vi "Read CJC Value.vi"(8 "error in (no error)":errorcluster, 11 "BNT_DMQmx-MCSV-TC in":refnum<class "BNT_DMQmx-MCSV-TC.lvclass">) -> (0 "error out":errorcluster, 2 "CJC Value":dbl=25.0 format="%0.2f", 3 "BNT_DMQmx-MCSV-TC out":refnum<class "BNT_DMQmx-MCSV-TC.lvclass">)   [LabVIEW 2016, in "BNT_DAQmx.lvlib" / "BNT_DMQmx-MCSV-TC.lvclass"]
doc: "Read CJC Value."
uses:
  BNT_DMQmx-MCSV-TC.lvclass
  BNT_DMQmx-MCSV-TC.lvclass/BNT_DMQmx-MCSV-TC.ctl
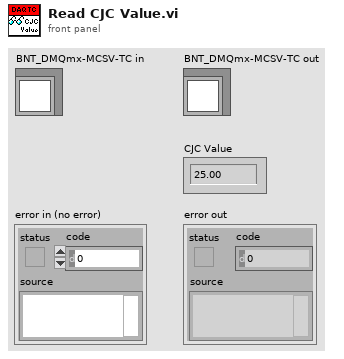
[diagram p1: front panel]
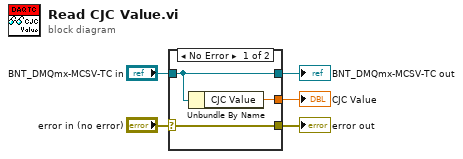
[diagram p0: block diagram]
diagram:
  n1 = case shown="No Error" "error in (no error)" {
    selector: "error in (no error)" -> [w8 w9]
    tunnel: [w8 w9] -> w4
    tunnel: [w7 w10] -> w2
    tunnel: "BNT_DMQmx-MCSV-TC in" -> [w7 w10]
    tunnel: [w6 _] -> w1
    frame No Error {
      n2 = Unbundle By Name(w7) -> ("CJC Value"=w6:dbl)
    }
    frame Error {
    }
  }
  "error out" <- w4
  "BNT_DMQmx-MCSV-TC out" <- w2
  "CJC Value" <- w1
